vi "read_out_equipment.vi"   [LabVIEW 2016]
uses:
  Global Variables/global.vi
  Instrument_Setup.vi
  Global Variables/Data_Display_global.vi
types:
  T1 = typedef "20TVTI_Cluster.ctl" = cluster{"Temperatur (K)":dbl, "Setpoint (K)":dbl, "Rate (K/min)":dbl, "Heater (%)":dbl, "NV (%)":dbl, "Heater Manual":bool, "NV Manual":bool, "Go to Set":bool, "Pressure":dbl, "Heater SP":dbl, "Valid?":bool, "Set Heater SP":bool, "Set NV SP":bool, "Heater (%) Display":dbl, "NV (%) Display":dbl, "NV Setpoint":dbl, "Change Heater Status":bool, "Change NV Status":bool, "Change Sweep Type":bool}
  T2 = typedef "VTI-cluster.ctl" = cluster{"Temperatur (K)":dbl, "Setpoint (K)":dbl, "Rate (K/min)":dbl, "Heater (%)":dbl, "NV (%)":dbl, "Heater Manual":bool, "NV Manual":bool, "Go to Set":bool, "Pressure":dbl, "Heater SP":dbl, "Valid?":bool, "Set Heater SP":bool, "Set NV SP":bool, "Heater (%) Display":dbl, "NV (%) Display":dbl, "NV Setpoint":dbl, "Change Heater Status":bool, "Change NV Status":bool, "Sample 3":dbl, "Sample 2":dbl, "Sweep-State":bool, "Set Auto PID":bool, "Auto PID":bool, "Stopp":bool, "Setpoint-Sweep":dbl}
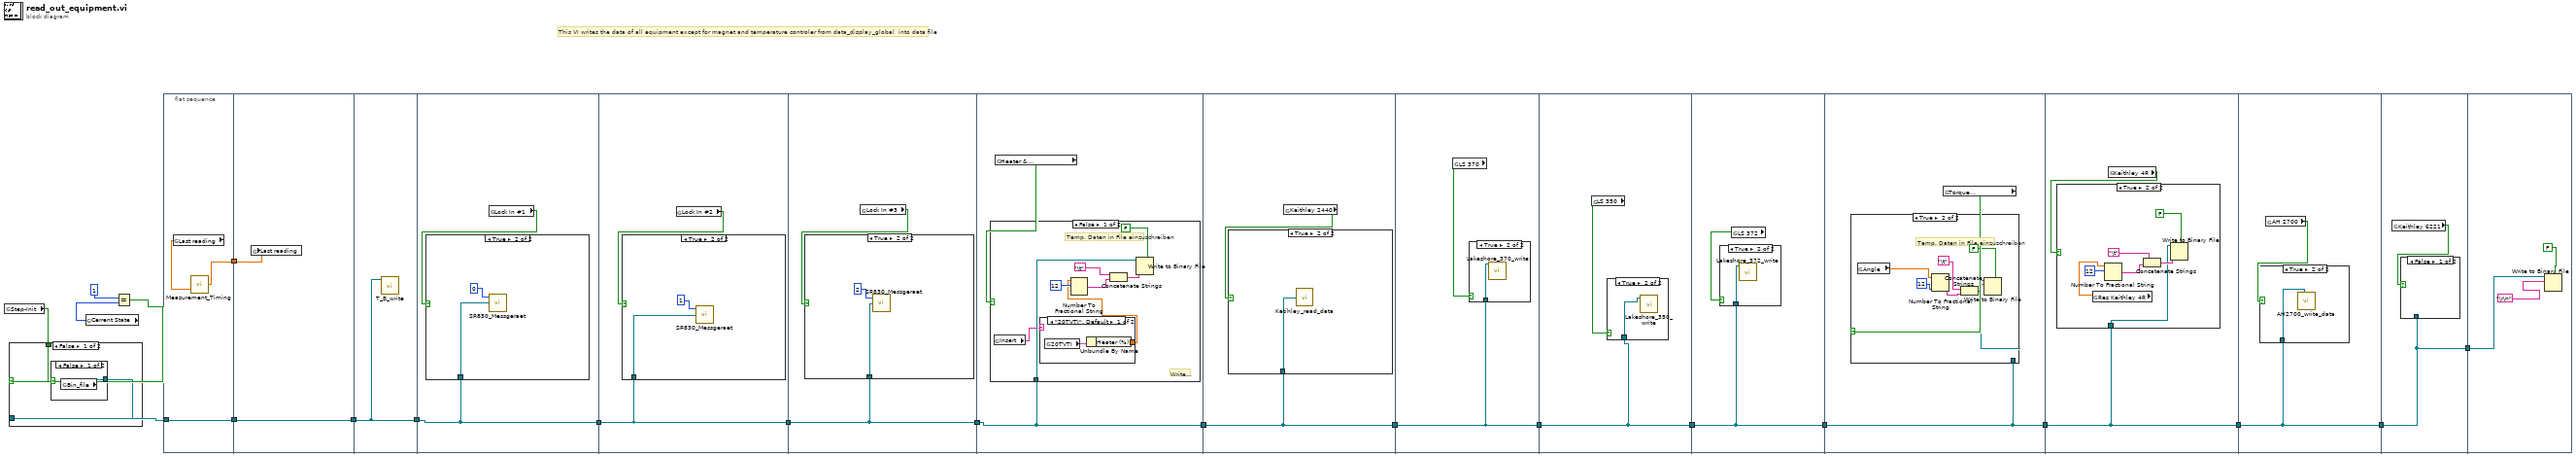
[diagram p0: block diagram]
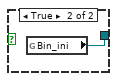
[diagram p2: hidden frame]
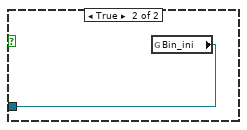
[diagram p3: hidden frame]
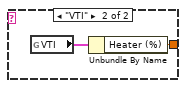
[diagram p7: hidden frame]
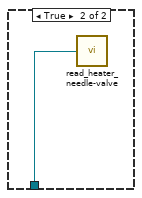
[diagram p8: hidden frame]
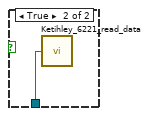
[diagram p16: hidden frame]
diagram:
  # "This VI writes the data of all equipment except for magnet and temperature controler from data_display_global  into data file"
  n1 = global read "global.vi" "Step-Init"() -> (w3:bool)
  n2 = global read "global.vi" "Cerrent State"() -> (w16:i32)
  n3 = Equal?(x=1, y=w16) -> (x = y?=w15:bool)
  n4 = case shown="False" w15 {
    tunnel: [w23 w26] -> w14
    tunnel: w3 -> [w22 _]
    frame False {
      n5 = case shown="False" w22 {
        tunnel: [w24 w25] -> w23
        frame False {
          n6 = global read "Instrument_Setup.vi" "Bin_file"() -> (w24:refnum<file>)
        }
        frame True {
          n7 = global read "Instrument_Setup.vi" "Bin_ini"() -> (w25:refnum<file>)
        }
      }
    }
    frame True {
      n8 = global read "Instrument_Setup.vi" "Bin_ini"() -> (w26:refnum<file>)
    }
  }
  n9 = flat-sequence {
    tunnel: w14 -> [w29]
    tunnel: [w29] -> w6
    tunnel: [w27] -> w4
    tunnel: w6 -> [w31]
    tunnel: [w31] -> w5
    tunnel: w4 -> [w30]
    tunnel: [w32] -> w8
    tunnel: w5 -> [w32]
    tunnel: [w33] -> w21
    tunnel: w8 -> [w33]
    tunnel: w21 -> [w37]
    tunnel: [w37] -> w20
    tunnel: w20 -> [w41]
    tunnel: [w41] -> w19
    tunnel: w19 -> [w45]
    tunnel: [w45] -> w18
    tunnel: w18 -> [w60]
    tunnel: [w60] -> w13
    tunnel: w13 -> [w63]
    tunnel: [w63] -> w2
    tunnel: w2 -> [w66]
    tunnel: [w66] -> w1
    tunnel: w1 -> [w69]
    tunnel: [w69] -> w10
    tunnel: w10 -> [w72]
    tunnel: [w72] -> w12
    tunnel: w12 -> [w81]
    tunnel: [w81] -> w11
    tunnel: w11 -> [w90]
    tunnel: [w90] -> w9
    tunnel: w9 -> [w93]
    tunnel: [w93] -> w7
    tunnel: w7 -> [w98]
    frame #0 {
      n10 = global read "Data_Display_global.vi" "Last reading"() -> (w28:dbl)
      n11 = call "Measurement_Timing.vi"("Last reading time"=w28) -> ("Last reading time out"=w27:dbl)  [unwired: 1 in]
    }
    frame #1 {
      n12 = global write "Data_Display_global.vi" "Last reading"(w30) -> ()
    }
    frame #2 {
      n13 = call "T_B_write.vi"("refnum"=w32) -> ()  [unwired: 6 in]
    }
    frame #3 {
      n14 = global read "Instrument_Setup.vi" "Lock In #1"() -> (w34:bool)
      n15 = case shown="True" w34 {
        tunnel: w33 -> [_ w35]
        frame False {
        }
        frame True {
          n16 = call "SR830_Messgeraet.vi"("refnum"=w35, "Numerisch"=0) -> ()  [unwired: 2 in]
        }
      }
    }
    frame #4 {
      n17 = global read "Instrument_Setup.vi" "Lock In #2"() -> (w38:bool)
      n18 = case shown="True" w38 {
        tunnel: w37 -> [_ w39]
        frame False {
        }
        frame True {
          n19 = call "SR830_Messgeraet.vi"("refnum"=w39, "Numerisch"=1) -> ()  [unwired: 2 in]
        }
      }
    }
    frame #5 {
      n20 = global read "Instrument_Setup.vi" "Lock In #3"() -> (w42:bool)
      n21 = case shown="True" w42 {
        tunnel: w41 -> [_ w43]
        frame False {
        }
        frame True {
          n22 = call "SR830_Messgeraet.vi"("refnum"=w43, "Numerisch"=2) -> ()  [unwired: 2 in]
        }
      }
    }
    frame #6 {
      n23 = global read "Instrument_Setup.vi" "Heater &\nNeedle Valve"() -> (w46:bool)
      n24 = case shown="False" w46 {
        tunnel: w45 -> [w49 w59]
        frame False {
          # "Temp. Daten in File einzuschreiben"
          # "Write File"
          n25 = global read "Instrument_Setup.vi" "Insert"() -> (w48:string)
          n26 = case shown="\"20TVTI\", Default" w48 {
            tunnel: [w55 w57] -> w47
            frame "20TVTI", Default {
              n27 = global read "Data_Display_global.vi" "20TVTI"() -> (w56:T1)
              n28 = Unbundle By Name(w56) -> ("Heater (%)"=w55:dbl)
            }
            frame "VTI" {
              n29 = global read "Data_Display_global.vi" "VTI"() -> (w58:T2)
              n30 = Unbundle By Name(w58) -> ("Heater (%)"=w57:dbl)
            }
          }
          n31 = Number To Fractional String(number=w47, precision (6)=i16 12) -> (F-format string=w52:string)  [unwired: 2 in]
          n32 = Concatenate Strings("\t", w52) -> (w54:string)
          n33 = Write to Binary File ("Write File")(file (use dialog)=w49, data=w54, 5:FALSE ("prepend array or string size? (T)")) -> ()  [unwired: 3 in, 3 out]
        }
        frame True {
          n34 = call "read_heater_needle-valve.vi"("refnum"=w59) -> ()
        }
      }
    }
    frame #7 {
      n35 = global read "Instrument_Setup.vi" "Keithley 2440"() -> (w61:bool)
      n36 = case shown="True" w61 {
        tunnel: w60 -> [_ w62]
        frame False {
        }
        frame True {
          n37 = call "Ketihley_read_data.vi"("refnum"=w62) -> ()
        }
      }
    }
    frame #8 {
      n38 = global read "Instrument_Setup.vi" "LS 370"() -> (w64:bool)
      n39 = case shown="True" w64 {
        tunnel: w63 -> [_ w65]
        frame False {
        }
        frame True {
          n40 = call "Lakeshore_370_write.vi"("File Reference"=w65) -> ()  [unwired: 5 in]
        }
      }
    }
    frame #9 {
      n41 = global read "Instrument_Setup.vi" "LS 350"() -> (w67:bool)
      n42 = case shown="True" w67 {
        tunnel: w66 -> [_ w68]
        frame False {
        }
        frame True {
          n43 = call "Lakeshore_350_write.vi"("File Reference"=w68) -> ()  [unwired: 5 in]
        }
      }
    }
    frame #10 {
      n44 = global read "Instrument_Setup.vi" "LS 372"() -> (w70:bool)
      n45 = case shown="True" w70 {
        tunnel: w69 -> [_ w71]
        frame False {
        }
        frame True {
          n46 = call "Lakeshore_372_write.vi"("File reference"=w71) -> ()  [unwired: 5 in]
        }
      }
    }
    frame #11 {
      n47 = global read "Instrument_Setup.vi" "Torque \nMeasurem."() -> (w73:bool)
      n48 = case shown="True" w73 {
        tunnel: w72 -> [_ w75]
        frame False {
        }
        frame True {
          # "Temp. Daten in File einzuschreiben"
          n49 = global read "Data_Display_global.vi" "Angle"() -> (w74:dbl)
          n50 = Number To Fractional String(number=w74, precision (6)=i16 12) -> (F-format string=w77:string)  [unwired: 2 in]
          n51 = Concatenate Strings("\t", w77) -> (w76:string)
          n52 = Write to Binary File ("Write File")(file (use dialog)=w75, data=w76, 5:FALSE ("prepend array or string size? (T)")) -> ()  [unwired: 3 in, 3 out]
        }
      }
    }
    frame #12 {
      n53 = global read "Instrument_Setup.vi" "Keithley 4R"() -> (w82:bool)
      n54 = case shown="True" w82 {
        tunnel: w81 -> [_ w83]
        frame False {
        }
        frame True {
          n55 = global read "Data_Display_global.vi" "Res Keithley 4R"() -> (w84:dbl)
          n56 = Number To Fractional String(number=w84, precision (6)=i16 12) -> (F-format string=w87:string)  [unwired: 2 in]
          n57 = Concatenate Strings("\t", w87) -> (w89:string)
          n58 = Write to Binary File ("Write File")(file (use dialog)=w83, data=w89, 5:FALSE ("prepend array or string size? (T)")) -> ()  [unwired: 3 in, 3 out]
        }
      }
    }
    frame #13 {
      n59 = global read "Instrument_Setup.vi" "AH 2700"() -> (w91:bool)
      n60 = case shown="True" w91 {
        tunnel: w90 -> [_ w92]
        frame False {
        }
        frame True {
          n61 = call "AH2700_write_data.vi"("File reference"=w92) -> ()  [unwired: 11 in]
        }
      }
    }
    frame #14 {
      n62 = global read "Instrument_Setup.vi" "Keithley 6221"() -> (w94:bool)
      n63 = case shown="False" w94 {
        tunnel: w93 -> [_ w95]
        frame False {
        }
        frame True {
          n64 = call "Ketihley_6221_read_data.vi"("refnum"=w95) -> ()
        }
      }
    }
    frame #15 {
      n65 = Write to Binary File ("Write File")(file (use dialog)=w98, data="\r\n", 5:FALSE) -> ()  [unwired: 3 in, 3 out]
    }
  }
